vi "Get Model Information.vi"(8 "error in":errorcluster, 11 "Alicat Device in":refnum<class "Alicat Device.lvclass">) -> (0 "error out":errorcluster, 1 "ModelOut":string, 2 "DataOut":string, 3 "Alicat Device out":refnum<class "Alicat Device.lvclass">)   [LabVIEW 2018, in "Alicat Lib.lvlib" / "Alicat Device.lvclass"]
doc: "Retrieve the model data from the Alicat device using the command <b>X??M*</b> where <b>X</b> is the address of the device. The model data will contain all the information to determine what the device is. This includes the scale, units and model."
uses:
  Alicat Device.lvclass
  Alicat Device.lvclass/Alicat Device.ctl
  reusable/Session APIs/Serial/Public/Asynchronous Write.vi
  reusable/Session APIs/Serial/Public/Get Multiline Strin.vi
  reusable/Session APIs/Serial/Serial Session.lvclass
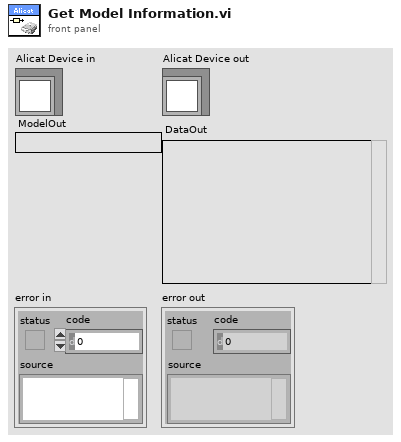
[diagram p1: front panel]
types:
  T1 = typedef "Serial Session.lvclass/Session Handle.ctl" = refnum<data-value>
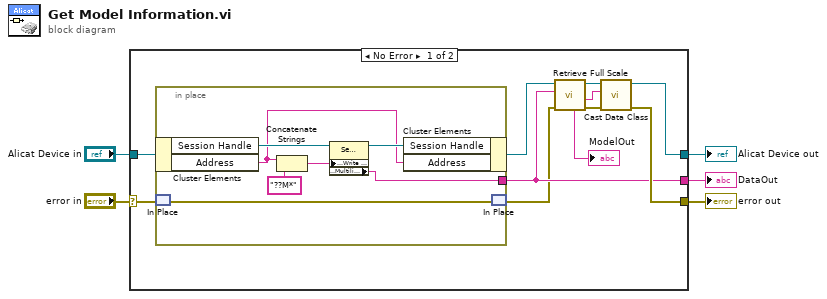
[diagram p0: block diagram]
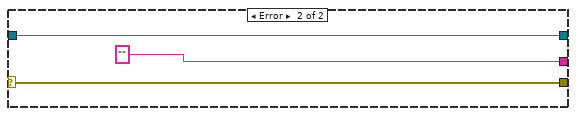
[diagram p2: hidden frame]
diagram:
  n1 = case shown="No Error" "error in" {
    selector: "error in" -> [w15 w26]
    tunnel: "Alicat Device in" -> [w16 w25]
    tunnel: [w14 w26] -> w2
    tunnel: [w13 w25] -> w4
    tunnel: [w12 "" ("DataOut")] -> w1
    frame No Error {
      n2 = in-place {
        in-place-border: [w21] -> w12
        n3 = in-place-cluster #1(w16) -> ("Session Handle"=w22:T1, "Address"=w19:string)
        n4 = in-place-match #2(w15) -> (w20:errorcluster)
        n5 = Concatenate Strings(w19, "??M*" ("string")) -> (w17:string)
        n6 = property class="Serial Session"(reference=w22, "Public:Write - Asynchronous"=w17) -> (reference out=w23:T1, "Public:Multiline Str"=w21:string)  [unwired: 1 in, 1 out]
        n7 = in-place-cluster #1("Session Handle"=w23, "Address"=w19) -> (w11:refnum<class "Alicat Device.lvclass">)
        n8 = in-place-match #2(w20) -> (w9:errorcluster)
      }
      n9 = call "Retrieve Full Scale.vi"("error in"=w9, "Model Data"=w12, "Alicat Device in"=w11) -> ("error out"=w8:errorcluster, "Type"=w7:string, "Alicat Device out"=w10:refnum<class "Alicat Device.lvclass">, "ModelOut"=→"ModelOut":string)  [unwired: 4 in, 1 out]
      n10 = call "Cast Data Class.vi"("error in"=w8, "Type"=w7, "Alicat Device in"=w10) -> ("error out"=w14:errorcluster, "Alicat Device out"=w13:refnum<class "Alicat Device.lvclass">)  [unwired: 6 in, 1 out]
    }
    frame Error {
    }
  }
  "error out" <- w2
  "Alicat Device out" <- w4
  "DataOut" <- w1
